vi "Text_Write To Clipboard.vi"(8 "Error":errorcluster, 11 "Test":string) -> (0 "Error Out":errorcluster)   [LabVIEW 2021]
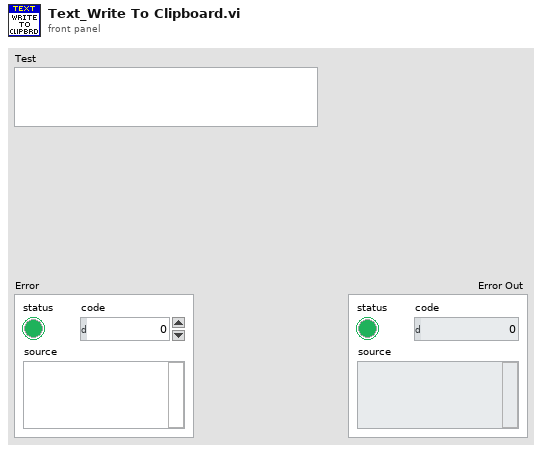
[diagram p1: front panel]
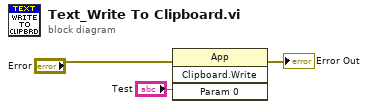
[diagram p0: block diagram]
diagram:
  n1 = invoke class="App" method="Clipboard.Write"(error in="Error", "Param 0"="Test") -> (error out=→"Error Out":errorcluster)  [unwired: 2 in, 3 out]
